vi "Write Poll Rate.vi"(8 "error in (no error)":errorcluster, 10 "Poll Rate":i64, 11 "Timed Loop Controller in":refnum<class "Timed Loop Controller.lvclass">) -> (0 "error out":errorcluster, 3 "Timed Loop Controller out":refnum<class "Timed Loop Controller.lvclass">)   [LabVIEW 2015, in "Timed Loop Controller.lvlib" / "Timed Loop Controller.lvclass"]
uses:
  Timed Loop Controller.lvclass
  Timed Loop Controller.lvclass/Timed Loop Controller.ctl
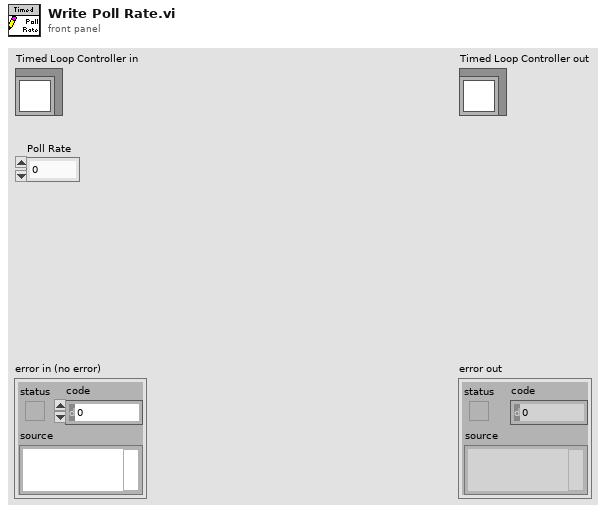
[diagram p1: front panel]
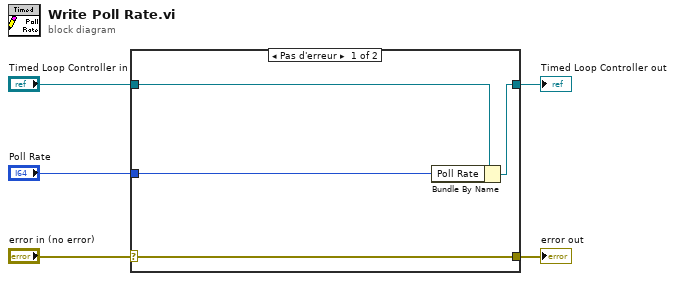
[diagram p0: block diagram]
diagram:
  n1 = case shown="Pas d'erreur" "error in (no error)" {
    selector: "error in (no error)" -> [w9 w10]
    tunnel: [w9 w10] -> w4
    tunnel: [w7 w11] -> w2
    tunnel: "Timed Loop Controller in" -> [w8 w11]
    tunnel: "Poll Rate" -> [w6 _]
    frame No Error {
      n2 = Bundle By Name(cluster=w8, "Poll Rate"=w6) -> (w7:refnum<class "Timed Loop Controller.lvclass">)
    }
    frame Error {
    }
  }
  "error out" <- w4
  "Timed Loop Controller out" <- w2
